vi "Re_sampling_1SS.vi"(11 "Waveform_main":waveform(sgl)) -> (3 "Waveform":waveform(dbl))   [LabVIEW 2017]
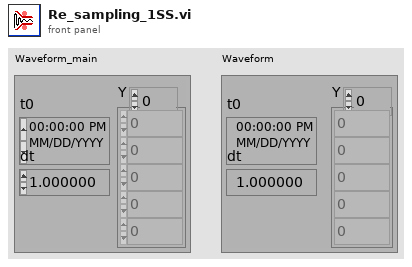
[diagram p1: front panel]
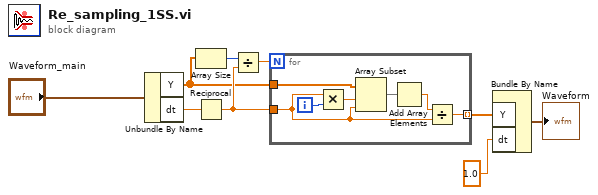
[diagram p0: block diagram]
diagram:
  n1 = Unbundle By Name("Waveform_main") -> ("Y"=w4:sgl[], "dt"=w1:dbl)
  n2 = Array Size(array=w4) -> (size(s)=w2:i32)
  n3 = Reciprocal(x=w1) -> (1/x=w5:dbl)
  n4 = Divide(x=w2, y=w5) -> (x/y=w3:dbl)
  n5 = for {
    N: w3 -> [_]
    tunnel: w4 -> [w16]
    tunnel: w5 -> [w12]
    tunnel: [w11] -> w6 mode=indexing
    i -> [w15]
    n6 = Multiply(x=w12, y=w15) -> (x*y=w10:dbl)
    n7 = Array Subset(array=w16, index=w10, length=w12) -> (w14:sgl[])
    n8 = Add Array Elements(numeric array=w14) -> (sum=w13:sgl)
    n9 = Divide(x=w13, y=w12) -> (x/y=w11:dbl)
  }
  n10 = Bundle By Name("Y"=w6, "dt"=1.0) -> (→"Waveform":waveform(dbl))  [unwired: 1 in]
